vi "Execute SQL Query with Rows.vi"(5 "cache size (1)":i32=1 min=1, 6 "error in (no error)":errorcluster, 7 "cursor type":T3, 8 "SQL query":string, 9 "connection reference":T2) -> (0 "error out":errorcluster, 2 "rows affected":i32, 3 "recordset reference":T4)   [LabVIEW 2013]
doc: "This VI is similar to the execute query included with the database connectivity toolkit. However, the number of rows affected is not output by the default VI, so this VI was included as a static dependency in order to provide that required data, the number of rows affected.\n\nThe original VI is copywrite national instruments"
uses:
  <vilib>/addons/database/Recordset.llb/Rec ObjectReference.ctl
  <vilib>/addons/database/Connection.llb/Conn ObjectReference.ctl
  <vilib>/addons/database/Auxilliary.llb/DB Tools Cursor Type.ctl
  <vilib>/addons/database/Recordset.llb/Rec DataMembers.ctl
  <vilib>/addons/database/_DB Variant To Data/Database Variant To Data.xnode
  <vilib>/addons/database/NI_Database_API.lvlib
panel:
  in  "default":T1
  in  "ADODB._Recordset":refnum<k7>
  in  "default data":T1
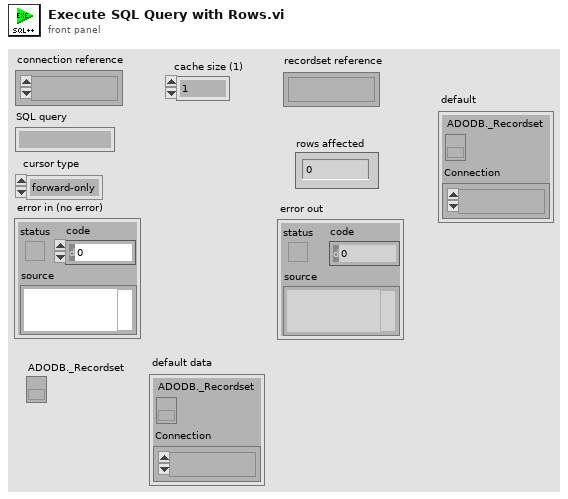
[diagram p1: front panel]
types:
  T1 = typedef "NI_Database_API.lvlib/Rec DataMembers.ctl" = cluster{"ADODB._Recordset":refnum<k7>, "Connection":T2}
  T2 = typedef "NI_Database_API.lvlib/Conn ObjectReference.ctl" = refnum<k1>
  T3 = typedef "NI_Database_API.lvlib/DB Tools Cursor Type.ctl" = enum16{"forward-only", "keyset", "dynamic", "static"}
  T4 = typedef "NI_Database_API.lvlib/Rec ObjectReference.ctl" = refnum<k1>
  T5 = typedef "NI_Database_API.lvlib/Conn DataMembers.ctl" = cluster{"ADODB._Connection":refnum<k7>, "recordset objects":i32, "command objects":i32}
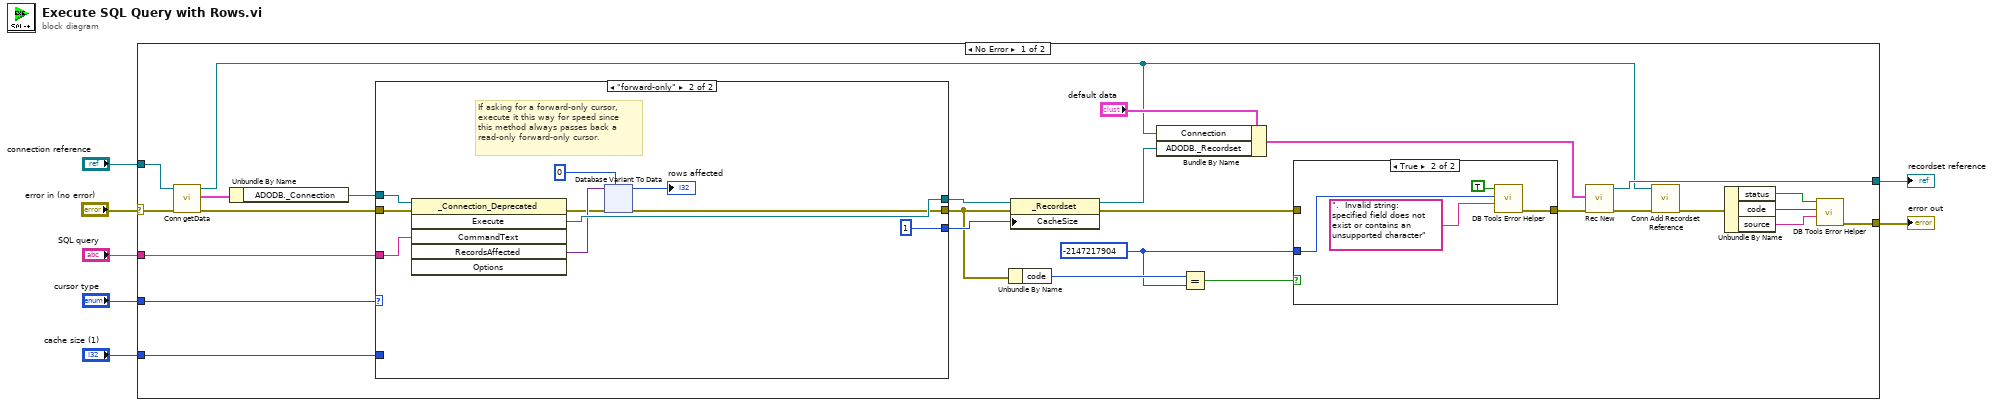
[diagram p0: block diagram]
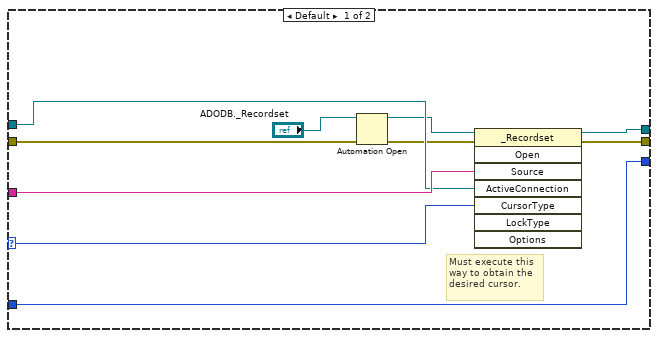
[diagram p3: hidden frame]
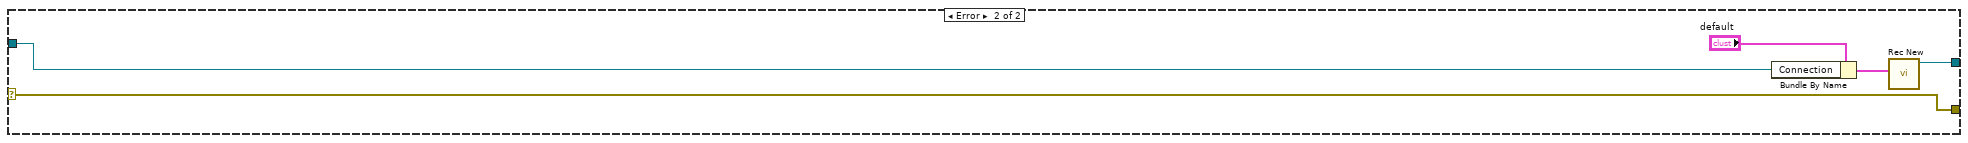
[diagram p4: hidden frame]
diagram:
  n1 = case shown="No Error" "error in (no error)" {
    selector: "error in (no error)" -> [w11 w96]
    tunnel: "cache size (1)" -> [w10 _]
    tunnel: [w32 w92] -> w1
    tunnel: "SQL query" -> [w30 _]
    tunnel: "cursor type" -> [w29 _]
    tunnel: "connection reference" -> [w26 w93]
    tunnel: [w13 w96] -> w3
    frame No Error {
      w19 = -2147217904
      n2 = call <vilib>:"Conn getData.vi"("error in (no error)"=w11, "connection reference"=w26) -> ("error out"=w25:errorcluster, "data"=w27:T5, "connection reference out"=w23:T2)  [unwired: 3 out]
      n3 = Unbundle By Name(w27) -> ("ADODB._Connection"=w24:refnum<k7>)
      n4 = case shown="\"forward-only\"" w29 {
        selector: w29 -> [w45 _]
        tunnel: w25 -> [w41 w58]
        tunnel: [w49 w57] -> w28
        tunnel: [w48 w50] -> w8
        tunnel: w30 -> [w47 w56]
        tunnel: w24 -> [w46 w59]
        tunnel: [w40 1 ("cache size (1)")] -> w9
        tunnel: w10 -> [w40 _]
        frame Default {
          # "Must execute this \nway to obtain the \ndesired cursor."
          n5 = Automation Open(error in (no error)=w41, Automation Refnum="ADODB._Recordset") -> (Automation Refnum=w43:refnum<k7>, error out=w42:errorcluster)  [unwired: 2 out]
          n6 = invoke class="_Recordset" method="Open"(reference=w43, error in=w42, "Source"=w47, "ActiveConnection"=w46, "CursorType"=w45) -> (reference out=w49:refnum<k7>, error out=w48:errorcluster)  [unwired: 3 in, 6 out]
        }
        frame "forward-only" {
          # "If asking for a forward-only cursor, \nexecute it this way for speed since \nthis method always passes back a \nread-only forward-only cursor."
          n7 = invoke class="_Connection_Deprecated" method="Execute"(reference=w59, error in=w58, "CommandText"=w56) -> (error out=w51:errorcluster, "Execute"=w57:refnum<k7>, "RecordsAffected"=w52:variant)  [unwired: 3 in, 3 out]
          n8 = xnode "Database Variant To Data"("database variant"=w52, "error in"=w51, "type"=0) -> ("data"=→"rows affected":i32, "error out"=w50:errorcluster)
        }
      }
      n9 = Unbundle By Name(w8) -> ("code"=w20:i32)
      n10 = property class="_Recordset"(reference=w28, error in=w8, "CacheSize"=w9) -> (reference out=w34:refnum<k7>, error out=w22:errorcluster)
      n11 = Bundle By Name(cluster="default data", "Connection"=w23, "ADODB._Recordset"=w34) -> (w12:T1)
      n12 = Equal?(x=w20, y=w19) -> (x = y?=w18:bool)
      n13 = case shown="True" w18 {
        tunnel: w22 -> [w35 _]
        tunnel: [w35 w39] -> w21
        tunnel: w19 -> [_ w37]
        frame False {
        }
        frame True {
          n14 = call <vilib>:"DB Tools Error Helper.vi"("source"=".  Invalid string: specified field does not exist or contains an unsupported character", "code"=w37, "status"=TRUE) -> ("error out"=w39:errorcluster)  [unwired: 1 in, 7 out]
        }
      }
      n15 = call <vilib>:"Rec New.vi"("error in (no error)"=w21, "initial data"=w12) -> ("error out"=w33:errorcluster, "recordset reference"=w32:T4)  [unwired: 4 out]
      n16 = call <vilib>:"Conn Add Recordset Reference.vi"("error in (no error)"=w33, "connection reference"=w23) -> ("error out"=w14:errorcluster)  [unwired: 9 out]
      n17 = Unbundle By Name(w14) -> ("status"=w16:bool, "code"=w15:i32, "source"=w17:string)
      n18 = call <vilib>:"DB Tools Error Helper.vi"("source"=w17, "code"=w15, "status"=w16) -> ("error out"=w13:errorcluster)  [unwired: 1 in, 7 out]
    }
    frame Error {
      n19 = Bundle By Name(cluster="default", "Connection"=w93) -> (w95:T1)
      n20 = call <vilib>:"Rec New.vi"("initial data"=w95) -> ("recordset reference"=w92:T4)  [unwired: 1 in, 5 out]
    }
  }
  "recordset reference" <- w1
  "error out" <- w3
